vi "AlliGator Compute G2_INTxMean(INT) Images.vi"(4 "INT Images":T1[](array[typedef]), 6 "Sum(INT)":T1, 7 "G2 Images":T1[](array[typedef]), 8 "Error In":errorcluster, 9 "Min(G2)":T1, 10 "Max(G2)":T1, 11 "Sum(G2)":T1) -> (0 "Error Out":errorcluster, 1 "Min(G2/INT*<INT>)":T1, 2 "Max(G2/INT*<INT>)":T1, 3 "Sum(G2/INT*<INT>)":T1, 5 "G2/INT*<INT> Images":T1[](array[typedef]))   [LabVIEW 2021, in "AlliGator Dual-Channel Datasets.lvlib"]
doc: "Computes G2/INT * <INT>."
uses:
  AlliGator Dual-Channel Datasets.lvlib
  <vilib>/vision/Image Controls.llb/IMAQ Image.ctl
  <vilib>/vision/NI_Vision_Development_Module.lvlib
  Image/Image.lvlib
  Utilities/Utilities.lvlib
panel:
  # "see the AlliGator License on the block diagram (Ctrl+E or Window:Show Block Diagram)"
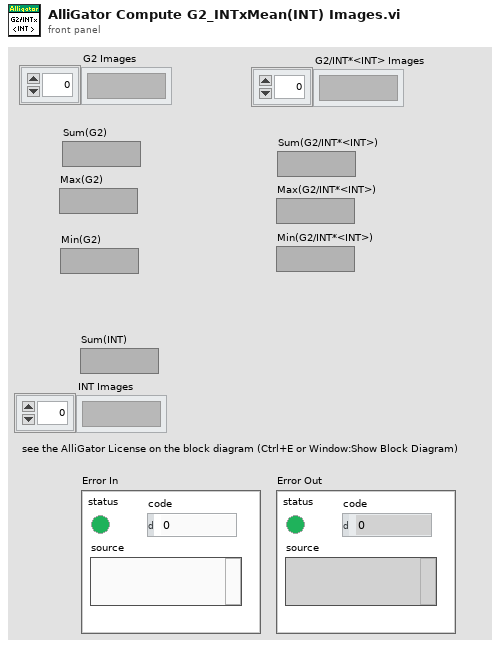
[diagram p1: front panel]
types:
  T1 = typedef "IMAQ Image.ctl" = refnum<image>
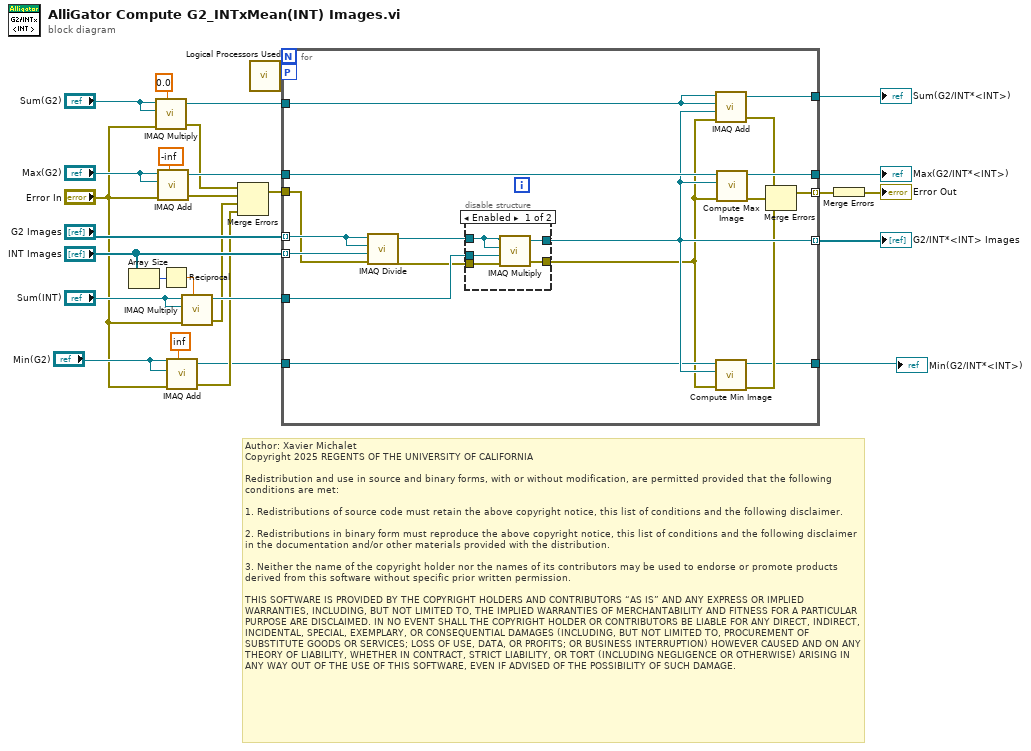
[diagram p0: block diagram]
diagram:
  # "Author: Xavier Michalet\nCopyright 2025 REGENTS OF THE UNIVERSITY OF CALIFORNIA\n\nRedistribution and use in source and binary forms, with or without modification, are permitted provided that the following conditions are met:\n\n1. Redistributions of source code must retain the above copyright notice, this list of conditions and the following disclaimer.\n\n2. Redistributions in binary form must reproduce the above copyright notice, this list of conditions and the following disclaimer in the documentation and/or other materials provided with the distribution.\n\n3. Neither the name of the copyright holder nor the names of its contributors may be used to endorse or promote products derived from this software without specific prior written permission.\n\nTHIS SOFTWARE IS PROVIDED BY THE COPYRIGHT HOLDERS AND CONTRIBUTORS “AS IS” AND ANY EXPRESS OR IMPLIED WARRANTIES, INCLUDING, BUT NOT LIMITED TO, THE IMPLIED WARRANTIES OF MERCHANTABILITY AND FITNESS FOR A PARTICULAR PURPOSE ARE DISCLAIMED. IN NO EVENT SHALL THE COPYRIGHT HOLDER OR CONTRIBUTORS BE LIABLE FOR ANY DIRECT, INDIRECT, INCIDENTAL, SPECIAL, EXEMPLARY, OR CONSEQUENTIAL DAMAGES (INCLUDING, BUT NOT LIMITED TO, PROCUREMENT OF SUBSTITUTE GOODS OR SERVICES; LOSS OF USE, DATA, OR PROFITS; OR BUSINESS INTERRUPTION) HOWEVER CAUSED AND ON ANY THEORY OF LIABILITY, WHETHER IN CONTRACT, STRICT LIABILITY, OR TORT (INCLUDING NEGLIGENCE OR OTHERWISE) ARISING IN ANY WAY OUT OF THE USE OF THIS SOFTWARE, EVEN IF ADVISED OF THE POSSIBILITY OF SUCH DAMAGE."
  n1 = Array Size(array="INT Images") -> (size(s)=w9:i32)
  n2 = call "IMAQ Multiply"("Image Src A"="Sum(G2)", "Constant"=0.0, "Image Dst"="Sum(G2)", "error in (no error)"="Error In") -> ("Image Dst Out"=w24:T1, "error out"=w17:errorcluster)  [unwired: 3 in]
  n3 = call "IMAQ Add"("Image Src A"="Max(G2)", "Constant"=-inf, "Image Dst"="Max(G2)", "error in (no error)"="Error In") -> ("Image Dst Out"=w28:T1, "error out"=w19:errorcluster)  [unwired: 3 in]
  n4 = Reciprocal(x=w9) -> (1/x=w8:dbl)
  n5 = call "IMAQ Add"("Image Src A"="Min(G2)", "Constant"=inf, "Image Dst"="Min(G2)", "error in (no error)"="Error In") -> ("Image Dst Out"=w2:T1, "error out"=w3:errorcluster)  [unwired: 3 in]
  n6 = call "IMAQ Multiply"("Image Src A"="Sum(INT)", "Constant"=w8, "Image Dst"="Sum(INT)", "error in (no error)"="Error In") -> ("Image Dst Out"=w12:T1, "error out"=w7:errorcluster)  [unwired: 3 in]
  n7 = Merge Errors(w17, w19, w7, w3) -> (w18:errorcluster)
  n8 = call "Logical Processors Used.vi"() -> ("# Logical Processor Used"=w14:i32)  [unwired: 6 in]
  n9 = for {
    tunnel: "INT Images" -> [w37] mode=indexing
    tunnel: "G2 Images" -> [w43] mode=indexing
    workers-P: w14 -> [_]
    tunnel: w28 -> [w46]
    tunnel: [w45] -> w20
    tunnel: [w44] -> w16 mode=indexing
    tunnel: w12 -> [w41]
    tunnel: [w33] -> w21 mode=indexing
    tunnel: w24 -> [w39]
    tunnel: [w38] -> w22
    tunnel: w18 -> [w34]
    tunnel: w2 -> [w31]
    tunnel: [w29] -> w1
    n10 = call "IMAQ Divide"("Image Src A"=w43, "Image Dst"=w43, "Image Src B"=w37, "error in (no error)"=w34) -> ("Image Dst Out"=w42:T1, "error out"=w40:errorcluster)  [unwired: 3 in]
    n11 = disable-structure shown="Enabled" {
      disable-tunnel: w42 -> [w51 w53]
      disable-tunnel: w41 -> [w50 _]
      disable-tunnel: w40 -> [w49 w52]
      disable-tunnel: [w48 w53] -> w33
      disable-tunnel: [w47 w52] -> w30
      frame Enabled {
        n12 = call "IMAQ Multiply"("Image Src A"=w51, "Image Dst"=w51, "Image Src B"=w50, "error in (no error)"=w49) -> ("Image Dst Out"=w48:T1, "error out"=w47:errorcluster)  [unwired: 3 in]
      }
      frame Disabled {
      }
    }
    n13 = call "IMAQ Add"("Image Src A"=w39, "Image Dst"=w39, "Image Src B"=w33, "error in (no error)"=w30) -> ("Image Dst Out"=w38:T1, "error out"=w35:errorcluster)  [unwired: 3 in]
    n14 = call "Compute Min Image.vi"("error in (no error)"=w30, "New Image"=w33, "Min Image Dst"=w31) -> ("error out"=w32:errorcluster, "Min Image"=w29:T1)  [unwired: 7 in]
    n15 = call "Compute Max Image.vi"("error in (no error)"=w30, "New Image"=w33, "Max Image Dst"=w46) -> ("error out"=w36:errorcluster, "Max Image"=w45:T1)  [unwired: 7 in]
    n16 = Merge Errors(w35, w36, w32) -> (w44:errorcluster)
  }
  "Sum(G2/INT*<INT>)" <- w22
  "G2/INT*<INT> Images" <- w21
  "Max(G2/INT*<INT>)" <- w20
  "Min(G2/INT*<INT>)" <- w1
  n17 = Merge Errors(w16) -> (→"Error Out":errorcluster)
